vi "return class.vi"() -> (0 "ClassOutsideProject.lvclass":refnum<class "ClassOutsideProject.lvclass">)   [LabVIEW 2023]
uses:
  ClassOutsideProject.lvclass
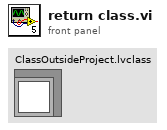
[diagram p1: front panel]
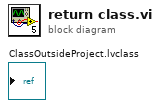
[diagram p0: block diagram]
diagram:
